vi "Get Results Format.vi"(8 "error IO":errorcluster, 11 "VISA resource name":refnum<visa-resource-name>) -> (0 "error Out":errorcluster, 2 "Results Displayed (2:Last)":u16(ring)=2 items=["All", "Pass / Fail", "Last"], 3 "VISA resource Out":refnum<visa-resource-name>)   [LabVIEW 2020, in "Associated Research 78XX Series.lvlib"]
uses:
  <instrlib>/Associated Research 78XX Series/Associated Research 78XX Series.lvlib
panel:
  # "0 - All\n1 - Pass/Fail\n2 - Last"
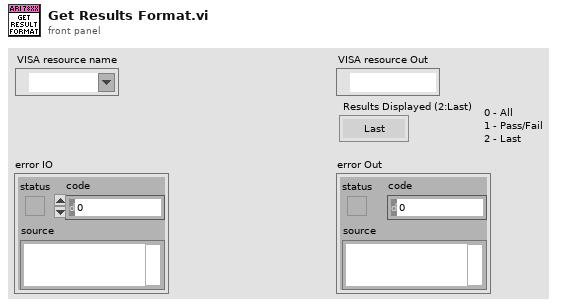
[diagram p1: front panel]
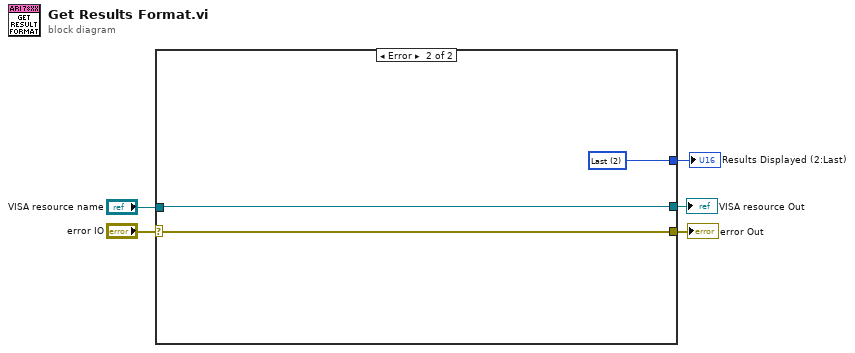
[diagram p0: block diagram]
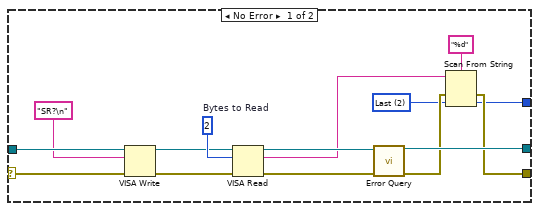
[diagram p2: hidden frame]
diagram:
  n1 = case shown="Error" "error IO" {
    selector: "error IO" -> [w20 w23]
    tunnel: [w8 w23] -> w2
    tunnel: [w18 w22] -> w3
    tunnel: "VISA resource name" -> [w19 w22]
    tunnel: [w7 w21] -> w1
    frame No Error {
      w6 = u16 2 items=["All", "Pass / Fail", "Last"] ("Results Displayed (2:Last)")
      w14 = u32 2  # Bytes to Read
      n2 = VISA Write(VISA resource name=w19, write buffer="SR?\n" ("Command to Send (empty)"), error in (no error)=w20) -> (VISA resource name out=w13:refnum<visa-resource-name>, error out=w12:errorcluster)  [unwired: 1 out]
      n3 = VISA Read(VISA resource name=w13, byte count=w14, error in (no error)=w12) -> (VISA resource name out=w16:refnum<visa-resource-name>, read buffer=w11:string, error out=w15:errorcluster)  [unwired: 1 out]
      n4 = call <instrlib>:"Error Query.vi"("VISA resource name"=w16, "error in (no error)"=w15) -> ("VISA resource name out"=w18:refnum<visa-resource-name>, "error out"=w9:errorcluster)  [unwired: 10 in, 2 out]
      n5 = Scan From String(format string="%d", input string=w11, error in=w9, default 1=w6) -> (error out=w8:errorcluster, output 1=w7:u16)  [unwired: 1 in, 2 out]
    }
    frame Error {
      w21 = u16 2 items=["All", "Pass / Fail", "Last"] ("Results Displayed (2:Last)")
    }
  }
  "VISA resource Out" <- w3
  "error Out" <- w2
  "Results Displayed (2:Last)" <- w1
